vi "SLSC Get SLSC name from Custom Device Ref.vi"(6 "connect timeout":dbl=5.0 format="%#_13g", 8 "error in (no error)":errorcluster, 9 "Wait for mDSN?":bool, 11 "Item Ref in":T1 format="%.0x") -> (0 "error out":errorcluster, 1 "SLSC Chassis Name":string, 2 "SLSC Module Name":string, 3 "Item Ref out":T1 format="%.0x")   [LabVIEW 2017, in "SLSC CD System Explorer.lvlib"]
uses:
  SLSC CD System Explorer.lvlib
  <vilib>/NI Veristand/Custom Device API/Custom Device Item Ref.ctl
  Shared/Constants.vi
  <vilib>/NI Veristand/Custom Device API/Get Item Property (U32).vi
  Shared/SLSC EDS Shared.lvlib
  <vilib>/NI VeriStand/Custom Device API/Custom Device API.lvlib
  SLSC CD Engine/SLSC CD Engine.lvlib
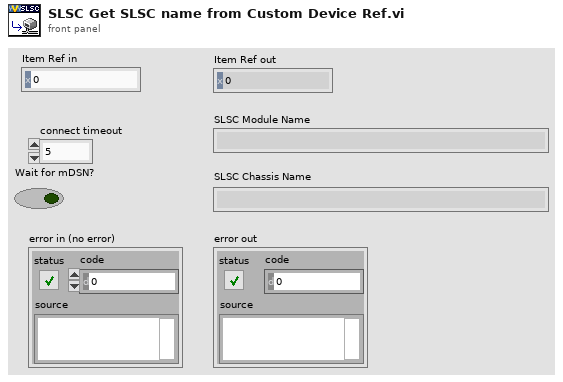
[diagram p1: front panel]
types:
  T1 = typedef "Custom Device API.lvlib/Custom Device Item Ref.ctl" = u64
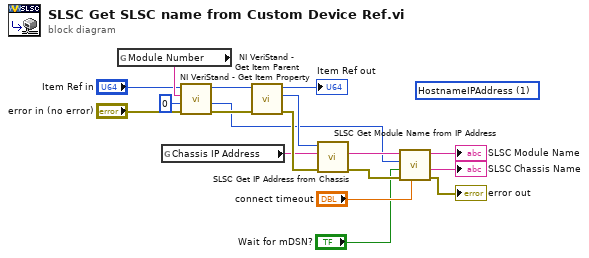
[diagram p0: block diagram]
diagram:
  (unwired) 1 items=["ChassisName", "HostnameIPAddress"] ("Chassis ID Type")
  n1 = global read "Constants.vi" "Module Number"() -> (w9:string)
  n2 = global read "Constants.vi" "Chassis IP Address"() -> (w12:string)
  n3 = call-poly <vilib>:"NI VeriStand - Get Item Property.vi"("error in (no error)"="error in (no error)", "Default Value"=u32 0, "Property Name"=w9, "Item Ref in"="Item Ref in") -> ("error out"=w7:errorcluster, "Value"=w3:u32, "Item Ref out"=w6:T1)  [unwired: 4 in, 1 out]
  n4 = call <vilib>:"NI VeriStand - Get Item Parent.vi"("error in (no error)"=w7, "Item Ref in"=w6) -> ("error out"=w14:errorcluster, "Parent Ref"=w13:T1, "Item Ref out"=→"Item Ref out":T1)  [unwired: 6 in, 1 out]
  n5 = call "SLSC Get IP Address from Chassis.vi"("error in (no error)"=w14, "IP Address Global Name"=w12, "Parent Ref"=w13) -> ("error out"=w17:errorcluster, "Name or IP Address"=w15:string)  [unwired: 5 in, 2 out]
  n6 = call "SLSC Get Module Name from IP Address.vi"("connect timeout"="connect timeout", "Error In"=w17, "Wait for mDSN?"="Wait for mDSN?", "Slot #"=w3, "Chassis IP Address"=w15) -> ("Error Out"=→"error out":errorcluster, "SLSC Chassis Name"=→"SLSC Chassis Name":string, "SLSC Module Name"=→"SLSC Module Name":string)  [unwired: 4 in]
